vi "总磷总氮测量数据储存.vi"   [LabVIEW 2016, in "斯坦道总氮.lvlib"]
types:
  T1 = enum16{"水样测试", "标样核查", "跨度核查", "零点核查", "加标回收", "空白测试", "平行样"}
  T2 = cluster{"时间标识":timestamp, "测量模式":enum16{"维护数据", "水样测试", "标样核查", "零点核查", "跨度核查", "空白测试", "平行样测试", "加标回收", "空白校准", "标样校准", "初始化（清洗）", "快捷测试"}, "数据标记表":string, "监测值":sgl, "单位":u16, "数据标识":string, "因子编码":u32, "标样参考值":sgl, "F0":sgl, "F1":sgl, "F2":sgl, "F3":sgl, "F4":sgl, "F5":sgl, "F6":sgl, "F7":sgl, "X":sgl, "温度":sgl, "湿度":sgl, "量程标识":string, "SN":string, "跨度值":sgl, "X1":sgl}
  T3 = enum16{"维护数据", "水样测试", "标样核查", "零点核查", "跨度核查", "空白测试", "平行样测试", "加标回收", "空白校准", "标样校准", "初始化（清洗）", "快捷测试"}
  T4 = enum16{"维护数据", "水样测试", "标样核查", "零点核查", "跨度核查", "空白测试", "平行样测试", "加标回收", "空白校准", "标样校准", "初始化（清洗）"}
  T5 = cluster{"系统时间":timestamp, "工作状态":u16, "测量模式":enum16{"待机", "连续模式", "周期模式", "定点模式", "受控模式", "手动模式"}, "告警代码":u16, "故障代码":u16, "日志代码":u16, "软件版本":u16, "F0":sgl, "F1":sgl, "F2":sgl, "F3":sgl, "T":sgl, "H":sgl, "id":u16, "flowid":u16, "量程":u16, "总磷控温温度1":sgl, "营养盐控温温度2":sgl, "ADC":sgl}
  T6 = cluster{"运行模式":enum16{"维护模式", "常规模式", "应急模式", "质控模式"}, "质控频次":enum16{"关闭", "每天", "星期一", "星期二", "星期三", "星期四", "星期五", "星期六", "星期日"}, "空白核查时间":u16, "跨度核查时间":u16, "测量间隔":u16}
  T7 = cluster{"因子编码":u32, "单位":u16, "标样参考值":sgl, "水样数据时间":timestamp, "水样实测值":sgl, "水样数据标识":string, "标样数据时间":timestamp, "标样实测值":sgl, "标样数据标识":string, "空白数据时间":timestamp, "空白实测值":sgl, "空白数据标识":string, "零点核查数据时间":timestamp, "零点核查实测值":sgl, "零点核查数据标识":string, "跨度核查数据时间":timestamp, "跨度核查实测值":sgl, "跨度核查数据标识":string, "加标回收数据时间":timestamp, "加标回收实测值":sgl, "加标回收数据标识":string, "平行样数据时间":timestamp, "平行样实测值":sgl, "平行样数据标识":string, "F0":sgl, "F1":sgl, "F2":sgl, "F3":sgl, "F4":sgl, "F5":sgl, "F6":sgl, "F7":sgl, "温度":sgl, "湿度":sgl, "X值":sgl, "fidrange":u16, "X1值":sgl}[]
  T8 = cluster{"因子编码":u32, "单位":u16, "标样参考值":sgl, "水样数据时间":timestamp, "水样实测值":sgl, "水样数据标识":string, "标样数据时间":timestamp, "标样实测值":sgl, "标样数据标识":string, "空白数据时间":timestamp, "空白实测值":sgl, "空白数据标识":string, "零点核查数据时间":timestamp, "零点核查实测值":sgl, "零点核查数据标识":string, "跨度核查数据时间":timestamp, "跨度核查实测值":sgl, "跨度核查数据标识":string, "加标回收数据时间":timestamp, "加标回收实测值":sgl, "加标回收数据标识":string, "平行样数据时间":timestamp, "平行样实测值":sgl, "平行样数据标识":string, "F0":sgl, "F1":sgl, "F2":sgl, "F3":sgl, "F4":sgl, "F5":sgl, "F6":sgl, "F7":sgl, "温度":sgl, "湿度":sgl, "X值":sgl, "fidrange":u16, "X1值":sgl}
  T9 = cluster{"总磷跨度值":dbl, "总磷零点标准液浓度":dbl, "总磷跨度标准液浓度":dbl, "总磷标准液标准浓度":dbl, "总氮跨度值":dbl, "总氮零点标准液浓度":dbl, "总氮跨度标准液浓度":dbl, "总氮标准液标准浓度":dbl, "COD跨度值":dbl, "COD零点标准液浓度":dbl, "COD跨度标准液浓度":dbl, "COD标准液标准浓度":dbl, "氨氮跨度值":dbl, "氨氮零点标准液浓度":dbl, "氨氮跨度标准液浓度":dbl, "氨氮标准液标准浓度":dbl, "磷酸盐跨度值":dbl, "磷酸盐零点标准液浓度":dbl, "磷酸盐跨度标准液浓度":dbl, "磷酸盐标准液标准浓度":dbl, "硝氮跨度值":dbl, "硝氮零点标准液浓度":dbl, "硝氮跨度标准液浓度":dbl, "硝氮标准液标准浓度":dbl, "亚硝氮跨度值":dbl, "亚硝氮零点标准液浓度":dbl, "亚硝氮跨度标准液浓度":dbl, "亚硝氮标准液标准浓度":dbl, "硫化物跨度值":dbl, "硫化物零点标准液浓度":dbl, "硫化物跨度标准液浓度":dbl, "硫化物标准液标准浓度":dbl, "硅酸盐跨度值":dbl, "硅酸盐零点标准液浓度":dbl, "硅酸盐跨度标准液浓度":dbl, "硅酸盐标准液标准浓度":dbl, "总磷零点标准液偏差":dbl, "总磷跨度标准液偏差":dbl, "总磷标准液标准偏差":dbl, "总氮零点标准液偏差":dbl, "总氮跨度标准液偏差":dbl, "总氮标准液标准偏差":dbl, "COD零点标准液偏差":dbl, "COD跨度标准液偏差":dbl, "COD标准液标准偏差":dbl, "氨氮零点标准液偏差":dbl, "氨氮跨度标准液偏差":dbl, "氨氮标准液标准偏差":dbl, "磷酸盐零点标准液偏差":dbl, "磷酸盐跨度标准液偏差":dbl, "磷酸盐标准液标准偏差":dbl, "硝氮零点标准液偏差":dbl, "硝氮跨度标准液偏差":dbl, "硝氮标准液标准偏差":dbl, "亚硝氮零点标准液偏差":dbl, "亚硝氮跨度标准液偏差":dbl, "亚硝氮标准液标准偏差":dbl, "硫化物零点标准液偏差":dbl, "硫化物跨度标准液偏差":dbl, "硫化物标准液标准偏差":dbl, "硅酸盐零点标准液偏差":dbl, "硅酸盐跨度标准液偏差":dbl, "硅酸盐标准液标准偏差":dbl, "氟化物跨度值":dbl, "氟化物零点标准液浓度":dbl, "氟化物跨度标准液浓度":dbl, "氟化物标准液标准浓度":dbl, "氟化物零点标准液偏差":dbl, "氟化物跨度标准液偏差":dbl, "氟化物标准液标准偏差":dbl}
  T10 = typedef "斯坦道总氮.lvlib/关键参数.ctl" = cluster{"测量量程":sgl, "测量检出限":sgl, "测量精度":sgl, "测量间隔":sgl, "消解温度":sgl, "消解时长":sgl, "三项式系数":sgl, "二次多项式系数":sgl, "曲线斜率":sgl, "曲线截距":sgl, "线性相关系数":sgl, "空白校准时间":timestamp, "标样校准时间":timestamp, "测量信号值":sgl, "稀释倍数":sgl, "空白标定系数":sgl, "量程系数":sgl}
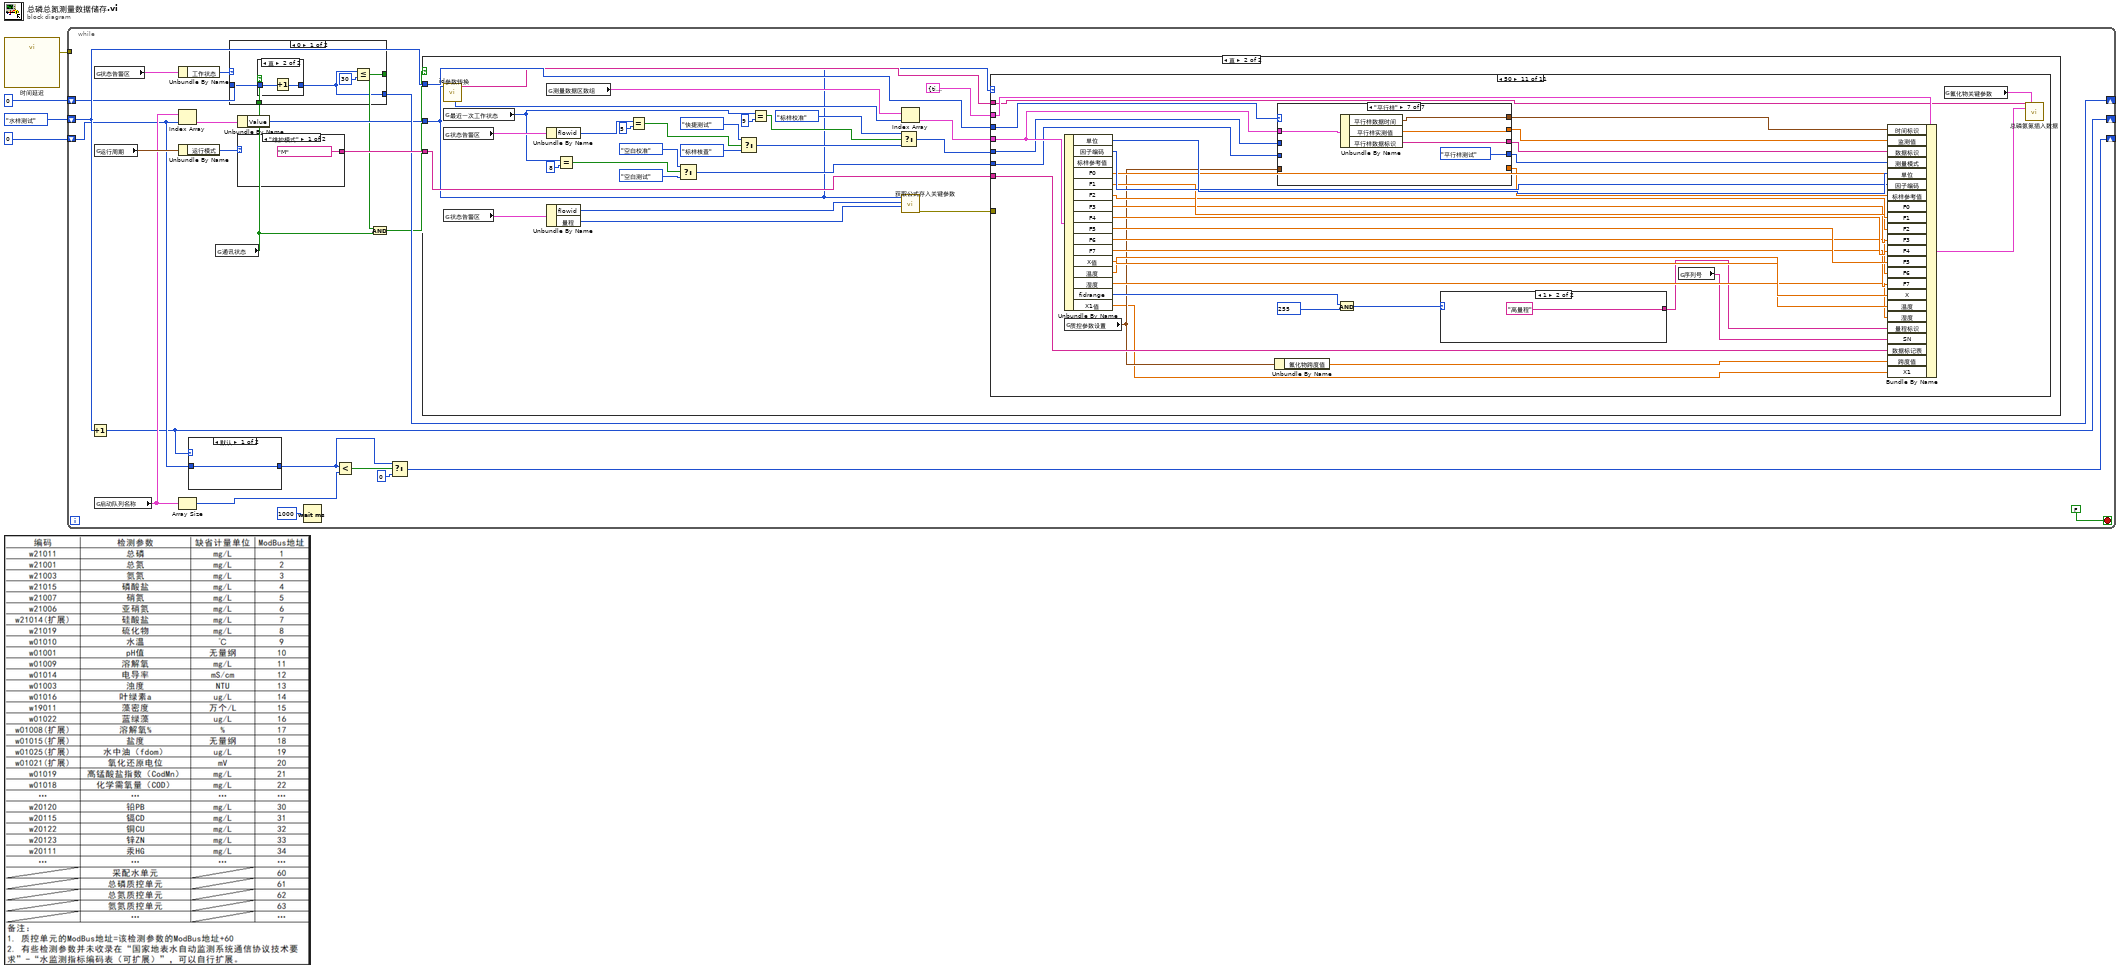
[diagram p0: block diagram]
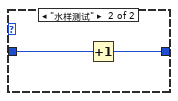
[diagram p2: hidden frame]
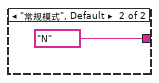
[diagram p5: hidden frame]
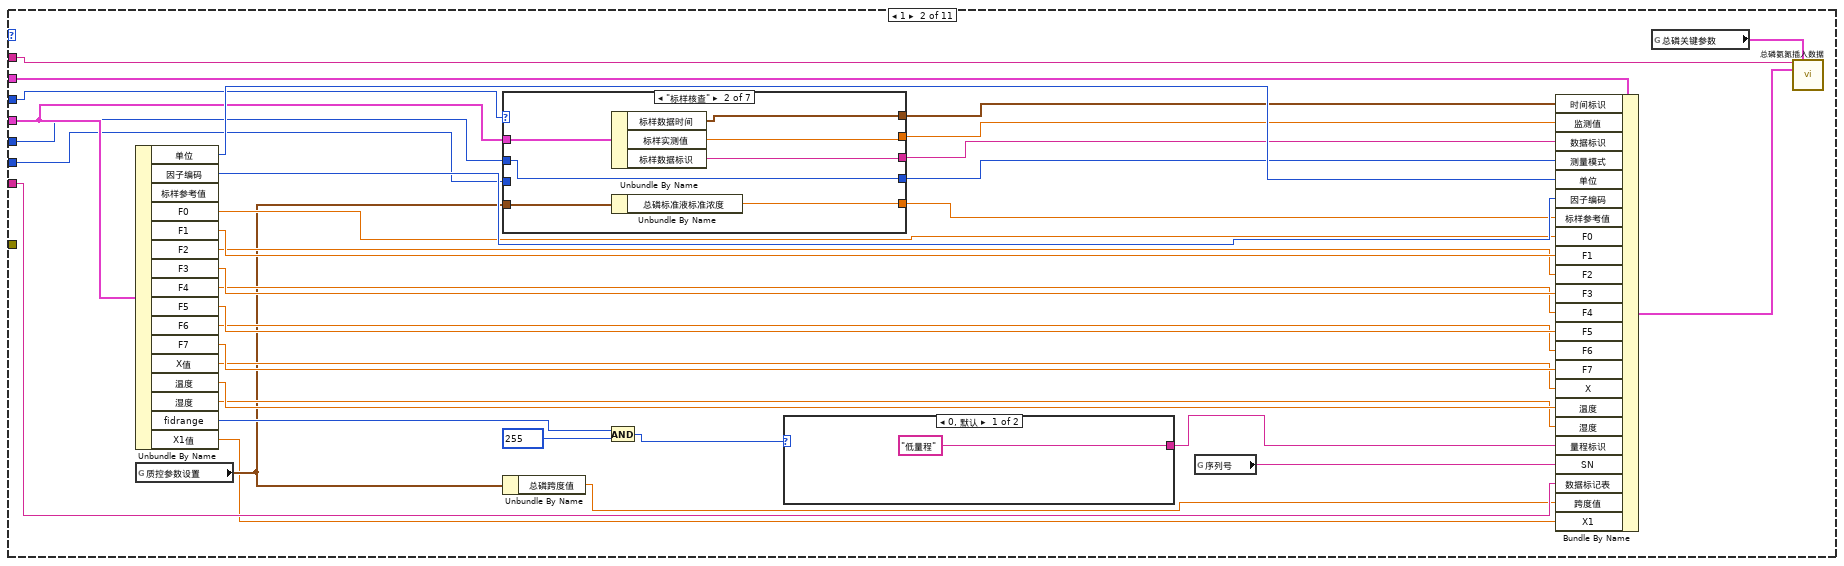
[diagram p8: hidden frame]
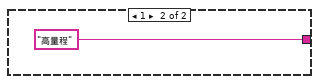
[diagram p9: hidden frame]
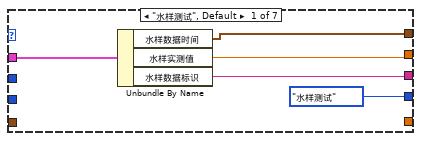
[diagram p10: hidden frame]
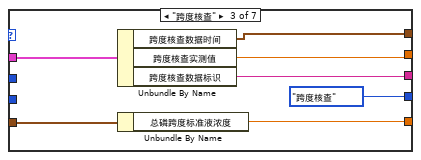
[diagram p11: hidden frame]
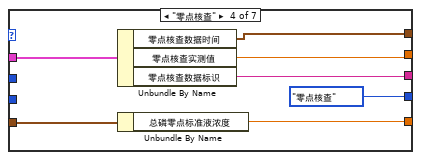
[diagram p12: hidden frame]
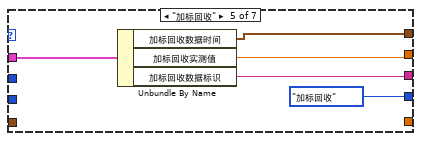
[diagram p13: hidden frame]
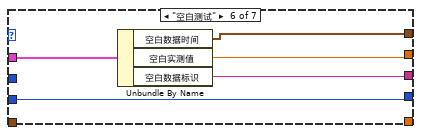
[diagram p14: hidden frame]
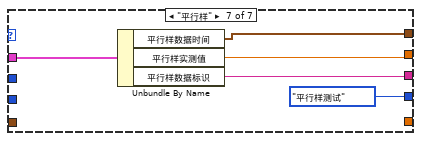
[diagram p15: hidden frame]
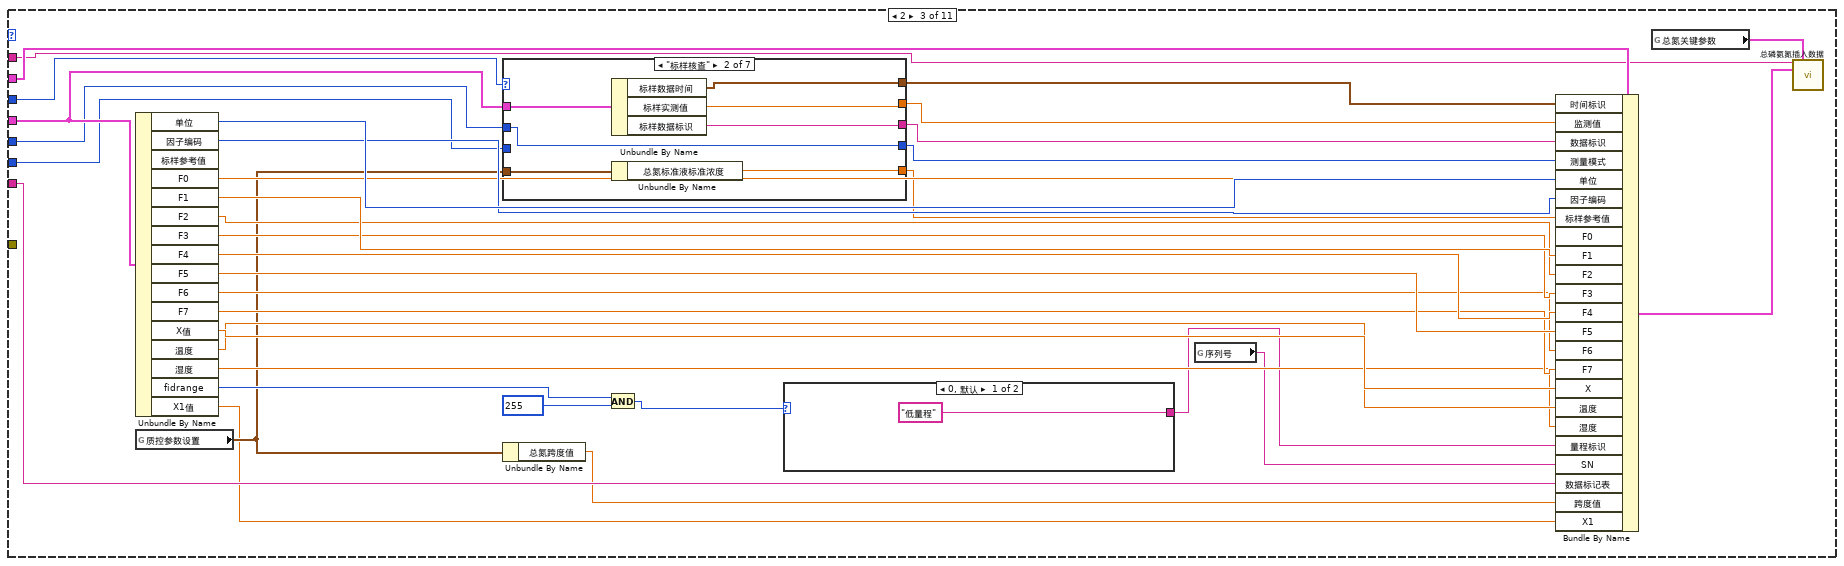
[diagram p16: hidden frame]
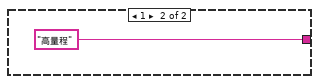
[diagram p17: hidden frame]
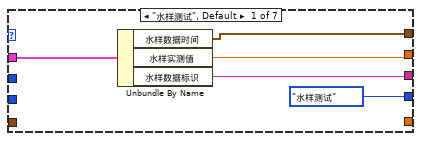
[diagram p18: hidden frame]
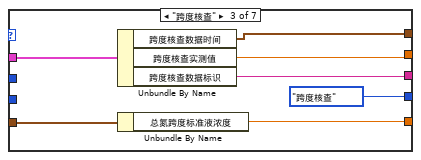
[diagram p19: hidden frame]
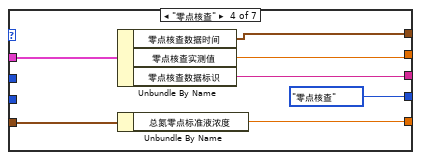
[diagram p20: hidden frame]
diagram:
  n1 = call "时间延迟"() -> ("error out"=w2:errorcluster)  [unwired: 11 in]
  n2 = while {
    shift-right: [w10] -> _
    shift-left: T1."水样测试" ("测量模式") -> [w25]
    shift-right: [w19] -> _
    shift-left: u32 0 ("等待时间（毫秒）") -> [w20]
    tunnel: w2 -> [_]
    shift-right: [w11] -> _
    shift-left: 0 -> [w14]
    stop <- FALSE stop-if-true
    n3 = Increment(x=w25) -> (x+1=w10:T1)
    n4 = global read "VAR总磷总氮全局变量.vi" "状态告警区"() -> (w22:T5)
    n5 = global read "总磷总氮断电保存全局变量.vi" "运行周期"() -> (w24:T6)
    n6 = global read "model config var.vi" "启动队列名称"() -> (w15:cluster{"String":string, "Value":u16}[])
    n7 = Unbundle By Name(w22) -> ("工作状态"=w21:u16)
    n8 = Index Array(array=w15, index=w14) -> (element=w17:cluster{"String":string, "Value":u16})
    n9 = Unbundle By Name(w24) -> ("运行模式"=w23:enum16{"维护模式", "常规模式", "应急模式", "质控模式"})
    n10 = Array Size(array=w15) -> (size(s)=w13:i32)
    n11 = case shown="默认" w10 {
      tunnel: w14 -> [w28 w30]
      tunnel: [w28 w29] -> w8
      frame Default {
      }
      frame "水样测试" {
        n12 = Increment(x=w30) -> (x+1=w29:i32)
      }
    }
    n13 = global read "VAR总磷总氮全局变量.vi" "通讯状态"() -> (w5:bool)
    n14 = case shown="0" w21 {
      tunnel: w20 -> [w35 _]
      tunnel: [w34 _] -> w19
      tunnel: [w32 _] -> w7
      tunnel: w5 -> [w31 _]
      frame 0 {
        n15 = case shown="真" w31 {
          tunnel: w35 -> [_ w37]
          tunnel: [_ w36] -> w34
          frame False {
          }
          frame True {
            n16 = Increment(x=w37) -> (x+1=w36:u32)
          }
        }
        n17 = Less Or Equal?(x=w34, y=u32 30) -> (x <= y?=w32:bool)
      }
      frame 1, Default {
      }
    }
    n18 = Unbundle By Name(w17) -> ("Value"=w16:u16)
    n19 = case shown="\"维护模式\"" w23 {
      tunnel: ["M" ("数据标记表") "N" ("数据标记表")] -> w26
      frame "维护模式" {
      }
      frame "常规模式", Default {
      }
    }
    n20 = Wait (ms)(milliseconds to wait=u32 1000 ("等待时间（毫秒）")) -> ()  [unwired: 1 out]
    n21 = Less?(x=w8, y=w13) -> (x < y?=w12:bool)
    n22 = And(x=w7, y=w5) -> (x .and. y?=w6:bool)
    n23 = Select(t=w8, s=w12, f=0) -> (s? t:f=w11:i32)
    n24 = case shown="真" w6 {
      tunnel: w26 -> [_ w68]
      tunnel: w25 -> [_ w67]
      tunnel: w16 -> [_ w40]
      frame False {
      }
      frame True {
        n25 = call "id参数转换.vi"("id"=w40) -> ("table输出"=w63:string, "数组资源索引"=w62:i32)  [unwired: 9 in]
        n26 = global read "VAR总磷总氮全局变量.vi" "最近一次工作状态"() -> (w54:u16)
        n27 = global read "VAR总磷总氮全局变量.vi" "状态告警区"() -> (w66:T5)
        n28 = global read "VAR总磷总氮全局变量.vi" "状态告警区"() -> (w44:T5)
        n29 = global read "VAR总磷总氮全局变量.vi" "测量数据区数组"() -> (w65:T7)
        n30 = Unbundle By Name(w66) -> ("flowid"=w51:u16)
        n31 = Unbundle By Name(w44) -> ("flowid"=w43:u16, "量程"=w42:u16)
        n32 = Equal?(x=w54, y=u16 8) -> (x = y?=w60:bool)
        n33 = Equal?(x=w51, y=u16 5) -> (x = y?=w49:bool)
        n34 = Select(t=T3."空白校准" ("测量模式"), s=w60, f=T3."空白测试" ("测量模式")) -> (s? t:f=w53:T3)
        n35 = Select(t=T3."快捷测试" ("测量模式"), s=w49, f=T3."标样核查" ("测量模式")) -> (s? t:f=w46:T3)
        n36 = Equal?(x=w54, y=u16 9) -> (x = y?=w56:bool)
        n37 = Select(t=T3."标样校准" ("测量模式"), s=w56, f=w46) -> (s? t:f=w52:T3)
        n38 = Index Array(array=w65, index=w62) -> (element=w64:T8)
        n39 = call "获取公式存入关键参数.vi"("量程"=w42, "flowid"=w43, "id"=w40) -> ("error out"=w41:errorcluster)  [unwired: 8 in]
        n40 = case shown="50" w40 {
          tunnel: w68 -> [_ w79 w157 w236 w314 w392 w470 w548 w626 w704 w782]
          tunnel: w67 -> [_ w87 w168 w246 w324 w402 w480 w558 w636 w714 w792]
          tunnel: T2 {"时间标识"=timestamp(0 s since 1904-01-01), "测量模式"=enum."水样测试", "数据标记表"="N", "监测值"=0.0, "单位"=0, "数据标识"="", "因子编码"=0, "标样参考值"=0.0, "F0"=0.0, "F1"=0.0, "F2"=0.0, "F3"=0.0, "F4"=0.0, "F5"=0.0, "F6"=0.0, "F7"=0.0, "X"=0.0, "温度"=0.0, "湿度"=0.0, "量程标识"="", "SN"="", "跨度值"=0.0, "X1"=0.0} ("data") -> [_ w77 w155 w234 w312 w390 w468 w546 w624 w702 w780]
          tunnel: w64 -> [_ w74 w152 w231 w309 w387 w465 w543 w621 w698 w776]
          tunnel: w63 -> [_ w73 w151 w229 w307 w385 w463 w541 w619 w697 w775]
          tunnel: w53 -> [_ w72 w150 w227 w306 w384 w462 w539 w618 w696 w774]
          tunnel: w52 -> [_ w71 w149 w228 w305 w383 w461 w540 w617 w695 w773]
          tunnel: w41 -> [_ _ _ _ _ _ _ _ _ _ _]
          frame Default {
          }
          frame 1 {
            n41 = Unbundle By Name(w74) -> ("单位"=w103:u16, "因子编码"=w102:u32, "F0"=w101:sgl, "F1"=w100:sgl, "F2"=w99:sgl, "F3"=w98:sgl, "F4"=w97:sgl, "F5"=w96:sgl, "F6"=w95:sgl, "F7"=w94:sgl, "X值"=w93:sgl, "温度"=w92:sgl, "湿度"=w91:sgl, "fidrange"=w85:u16, "X1值"=w69:sgl)  [unwired: 1 out]
            n42 = global read "总磷总氮断电保存全局变量.vi" "质控参数设置"() -> (w76:T9)
            n43 = case shown="\"标样核查\"" w87 {
              tunnel: w74 -> [w110 w117 w124 w131 w136 w141 w146]
              tunnel: [w109 w116 w123 w130 w135 w140 w145] -> w88
              tunnel: [w108 w115 w122 w129 w134 w139 w144] -> w89
              tunnel: [w107 w114 w121 w128 w133 w138 w143] -> w90
              tunnel: [T4."水样测试" ("测量模式") w111 T4."跨度核查" ("测量模式") T4."零点核查" ("测量模式") T4."加标回收" ("测量模式") w137 T4."平行样测试" ("测量模式")] -> w78
              tunnel: w76 -> [_ w113 w119 w126 _ _ _]
              tunnel: [_ w112 w118 w125 _ _ _] -> w86
              tunnel: w72 -> [_ _ _ _ _ w137 _]
              tunnel: w71 -> [_ w111 _ _ _ _ _]
              frame "水样测试", Default {
                n44 = Unbundle By Name(w110) -> ("水样数据时间"=w109:timestamp, "水样实测值"=w108:sgl, "水样数据标识"=w107:string)
              }
              frame "标样核查" {
                n45 = Unbundle By Name(w117) -> ("标样数据时间"=w116:timestamp, "标样实测值"=w115:sgl, "标样数据标识"=w114:string)
                n46 = Unbundle By Name(w113) -> ("总磷标准液标准浓度"=w112:dbl)
              }
              frame "跨度核查" {
                n47 = Unbundle By Name(w124) -> ("跨度核查数据时间"=w123:timestamp, "跨度核查实测值"=w122:sgl, "跨度核查数据标识"=w121:string)
                n48 = Unbundle By Name(w119) -> ("总磷跨度标准液浓度"=w118:dbl)
              }
              frame "零点核查" {
                n49 = Unbundle By Name(w131) -> ("零点核查数据时间"=w130:timestamp, "零点核查实测值"=w129:sgl, "零点核查数据标识"=w128:string)
                n50 = Unbundle By Name(w126) -> ("总磷零点标准液浓度"=w125:dbl)
              }
              frame "加标回收" {
                n51 = Unbundle By Name(w136) -> ("加标回收数据时间"=w135:timestamp, "加标回收实测值"=w134:sgl, "加标回收数据标识"=w133:string)
              }
              frame "空白测试" {
                n52 = Unbundle By Name(w141) -> ("空白数据时间"=w140:timestamp, "空白实测值"=w139:sgl, "空白数据标识"=w138:string)
              }
              frame "平行样" {
                n53 = Unbundle By Name(w146) -> ("平行样数据时间"=w145:timestamp, "平行样实测值"=w144:sgl, "平行样数据标识"=w143:string)
              }
            }
            n54 = Unbundle By Name(w76) -> ("总磷跨度值"=w75:dbl)
            n55 = And(x=w85, y=u16 255) -> (x .and. y?=w83:u16)
            n56 = case shown="0, 默认" w83 {
              tunnel: ["低量程" ("格式字符串") "高量程" ("格式字符串")] -> w82
              frame 0, Default {
              }
              frame 1 {
              }
            }
            n57 = global read "VAR总磷总氮全局变量.vi" "序列号"() -> (w80:string)
            n58 = Bundle By Name(cluster=w77, "时间标识"=w88, "监测值"=w89, "数据标识"=w90, "测量模式"=w78, "单位"=w103, "因子编码"=w102, "标样参考值"=w86, "F0"=w101, "F1"=w100, "F2"=w99, "F3"=w98, "F4"=w97, "F5"=w96, "F6"=w95, "F7"=w94, "X"=w93, "温度"=w92, "湿度"=w91, "量程标识"=w82, "SN"=w80, "数据标记表"=w79, "跨度值"=w75, "X1"=w69) -> (w81:T2)
            n59 = global read "VAR总磷总氮全局变量.vi" "总磷关键参数"() -> (w70:T10)
            n60 = call "总磷氨氮插入数据.vi"("table"=w73, "关键参数"=w70, "data"=w81) -> ()  [unwired: 12 in, 1 out]
          }
          frame 2 {
            n61 = Unbundle By Name(w152) -> ("单位"=w181:u16, "因子编码"=w180:u32, "F0"=w179:sgl, "F1"=w178:sgl, "F2"=w177:sgl, "F3"=w176:sgl, "F4"=w175:sgl, "F5"=w174:sgl, "F6"=w173:sgl, "F7"=w172:sgl, "X值"=w171:sgl, "温度"=w170:sgl, "湿度"=w169:sgl, "fidrange"=w161:u16, "X1值"=w147:sgl)  [unwired: 1 out]
            n62 = global read "总磷总氮断电保存全局变量.vi" "质控参数设置"() -> (w154:T9)
            n63 = case shown="\"标样核查\"" w168 {
              tunnel: w152 -> [w188 w195 w202 w209 w214 w219 w224]
              tunnel: [w187 w194 w201 w208 w213 w218 w223] -> w167
              tunnel: [w186 w193 w200 w207 w212 w217 w222] -> w166
              tunnel: [w185 w192 w199 w206 w211 w216 w221] -> w165
              tunnel: [T4."水样测试" ("测量模式") w189 T4."跨度核查" ("测量模式") T4."零点核查" ("测量模式") T4."加标回收" ("测量模式") w215 T4."平行样测试" ("测量模式")] -> w156
              tunnel: w154 -> [_ w191 w197 w204 _ _ _]
              tunnel: [_ w190 w196 w203 _ _ _] -> w164
              tunnel: w150 -> [_ _ _ _ _ w215 _]
              tunnel: w149 -> [_ w189 _ _ _ _ _]
              frame "水样测试", Default {
                n64 = Unbundle By Name(w188) -> ("水样数据时间"=w187:timestamp, "水样实测值"=w186:sgl, "水样数据标识"=w185:string)
              }
              frame "标样核查" {
                n65 = Unbundle By Name(w195) -> ("标样数据时间"=w194:timestamp, "标样实测值"=w193:sgl, "标样数据标识"=w192:string)
                n66 = Unbundle By Name(w191) -> ("总氮标准液标准浓度"=w190:dbl)
              }
              frame "跨度核查" {
                n67 = Unbundle By Name(w202) -> ("跨度核查数据时间"=w201:timestamp, "跨度核查实测值"=w200:sgl, "跨度核查数据标识"=w199:string)
                n68 = Unbundle By Name(w197) -> ("总氮跨度标准液浓度"=w196:dbl)
              }
              frame "零点核查" {
                n69 = Unbundle By Name(w209) -> ("零点核查数据时间"=w208:timestamp, "零点核查实测值"=w207:sgl, "零点核查数据标识"=w206:string)
                n70 = Unbundle By Name(w204) -> ("总氮零点标准液浓度"=w203:dbl)
              }
              frame "加标回收" {
                n71 = Unbundle By Name(w214) -> ("加标回收数据时间"=w213:timestamp, "加标回收实测值"=w212:sgl, "加标回收数据标识"=w211:string)
              }
              frame "空白测试" {
                n72 = Unbundle By Name(w219) -> ("空白数据时间"=w218:timestamp, "空白实测值"=w217:sgl, "空白数据标识"=w216:string)
              }
              frame "平行样" {
                n73 = Unbundle By Name(w224) -> ("平行样数据时间"=w223:timestamp, "平行样实测值"=w222:sgl, "平行样数据标识"=w221:string)
              }
            }
            n74 = Unbundle By Name(w154) -> ("总氮跨度值"=w153:dbl)
            n75 = And(x=w161, y=u16 255) -> (x .and. y?=w162:u16)
            n76 = case shown="0, 默认" w162 {
              tunnel: ["低量程" ("格式字符串") "高量程" ("格式字符串")] -> w160
              frame 0, Default {
              }
              frame 1 {
              }
            }
            n77 = global read "VAR总磷总氮全局变量.vi" "序列号"() -> (w158:string)
            n78 = Bundle By Name(cluster=w155, "时间标识"=w167, "监测值"=w166, "数据标识"=w165, "测量模式"=w156, "单位"=w181, "因子编码"=w180, "标样参考值"=w164, "F0"=w179, "F1"=w178, "F2"=w177, "F3"=w176, "F4"=w175, "F5"=w174, "F6"=w173, "F7"=w172, "X"=w171, "温度"=w170, "湿度"=w169, "量程标识"=w160, "SN"=w158, "数据标记表"=w157, "跨度值"=w153, "X1"=w147) -> (w159:T2)
            n79 = global read "VAR总磷总氮全局变量.vi" "总氮关键参数"() -> (w148:T10)
            n80 = call "总磷氨氮插入数据.vi"("table"=w151, "关键参数"=w148, "data"=w159) -> ()  [unwired: 12 in, 1 out]
          }
          frame 3 {
            n81 = Unbundle By Name(w231) -> ("单位"=w259:u16, "因子编码"=w258:u32, "F0"=w257:sgl, "F1"=w256:sgl, "F2"=w255:sgl, "F3"=w254:sgl, "F4"=w253:sgl, "F5"=w252:sgl, "F6"=w251:sgl, "F7"=w250:sgl, "X值"=w249:sgl, "温度"=w248:sgl, "湿度"=w247:sgl, "fidrange"=w239:u16, "X1值"=w225:sgl)  [unwired: 1 out]
            n82 = global read "总磷总氮断电保存全局变量.vi" "质控参数设置"() -> (w233:T9)
            n83 = case shown="\"空白测试\"" w246 {
              tunnel: w231 -> [w266 w273 w280 w287 w292 w297 w302]
              tunnel: [w265 w272 w279 w286 w291 w296 w301] -> w245
              tunnel: [w264 w271 w278 w285 w290 w295 w300] -> w244
              tunnel: [w263 w270 w277 w284 w289 w294 w299] -> w243
              tunnel: [T4."水样测试" ("测量模式") w267 T4."跨度核查" ("测量模式") T4."零点核查" ("测量模式") T4."加标回收" ("测量模式") w293 T4."平行样测试" ("测量模式")] -> w235
              tunnel: w233 -> [_ w269 w275 w282 _ _ _]
              tunnel: [_ w268 w274 w281 _ _ _] -> w242
              tunnel: w228 -> [_ w267 _ _ _ _ _]
              tunnel: w227 -> [_ _ _ _ _ w293 _]
              frame "水样测试", Default {
                n84 = Unbundle By Name(w266) -> ("水样数据时间"=w265:timestamp, "水样实测值"=w264:sgl, "水样数据标识"=w263:string)
              }
              frame "标样核查" {
                n85 = Unbundle By Name(w273) -> ("标样数据时间"=w272:timestamp, "标样实测值"=w271:sgl, "标样数据标识"=w270:string)
                n86 = Unbundle By Name(w269) -> ("氨氮标准液标准浓度"=w268:dbl)
              }
              frame "跨度核查" {
                n87 = Unbundle By Name(w280) -> ("跨度核查数据时间"=w279:timestamp, "跨度核查实测值"=w278:sgl, "跨度核查数据标识"=w277:string)
                n88 = Unbundle By Name(w275) -> ("氨氮跨度标准液浓度"=w274:dbl)
              }
              frame "零点核查" {
                n89 = Unbundle By Name(w287) -> ("零点核查数据时间"=w286:timestamp, "零点核查实测值"=w285:sgl, "零点核查数据标识"=w284:string)
                n90 = Unbundle By Name(w282) -> ("氨氮零点标准液浓度"=w281:dbl)
              }
              frame "加标回收" {
                n91 = Unbundle By Name(w292) -> ("加标回收数据时间"=w291:timestamp, "加标回收实测值"=w290:sgl, "加标回收数据标识"=w289:string)
              }
              frame "空白测试" {
                n92 = Unbundle By Name(w297) -> ("空白数据时间"=w296:timestamp, "空白实测值"=w295:sgl, "空白数据标识"=w294:string)
              }
              frame "平行样" {
                n93 = Unbundle By Name(w302) -> ("平行样数据时间"=w301:timestamp, "平行样实测值"=w300:sgl, "平行样数据标识"=w299:string)
              }
            }
            n94 = Unbundle By Name(w233) -> ("氨氮跨度值"=w232:dbl)
            n95 = And(x=w239, y=u16 255) -> (x .and. y?=w240:u16)
            n96 = case shown="0, 默认" w240 {
              tunnel: ["低量程" ("格式字符串") "高量程" ("格式字符串")] -> w238
              frame 0, Default {
              }
              frame 1 {
              }
            }
            n97 = global read "VAR总磷总氮全局变量.vi" "序列号"() -> (w237:string)
            n98 = Bundle By Name(cluster=w234, "时间标识"=w245, "监测值"=w244, "数据标识"=w243, "测量模式"=w235, "单位"=w259, "因子编码"=w258, "标样参考值"=w242, "F0"=w257, "F1"=w256, "F2"=w255, "F3"=w254, "F4"=w253, "F5"=w252, "F6"=w251, "F7"=w250, "X"=w249, "温度"=w248, "湿度"=w247, "量程标识"=w238, "SN"=w237, "数据标记表"=w236, "跨度值"=w232, "X1"=w225) -> (w230:T2)
            n99 = global read "VAR总磷总氮全局变量.vi" "氨氮关键参数"() -> (w226:T10)
            n100 = call "总磷氨氮插入数据.vi"("table"=w229, "关键参数"=w226, "data"=w230) -> ()  [unwired: 12 in, 1 out]
          }
          frame 4 {
            n101 = Unbundle By Name(w309) -> ("单位"=w337:u16, "因子编码"=w336:u32, "F0"=w335:sgl, "F1"=w334:sgl, "F2"=w333:sgl, "F3"=w332:sgl, "F4"=w331:sgl, "F5"=w330:sgl, "F6"=w329:sgl, "F7"=w328:sgl, "X值"=w327:sgl, "温度"=w326:sgl, "湿度"=w325:sgl, "fidrange"=w317:u16, "X1值"=w303:sgl)  [unwired: 1 out]
            n102 = global read "总磷总氮断电保存全局变量.vi" "质控参数设置"() -> (w311:T9)
            n103 = case shown="\"标样核查\"" w324 {
              tunnel: w309 -> [w344 w351 w358 w365 w370 w375 w380]
              tunnel: [w343 w350 w357 w364 w369 w374 w379] -> w323
              tunnel: [w342 w349 w356 w363 w368 w373 w378] -> w322
              tunnel: [w341 w348 w355 w362 w367 w372 w377] -> w321
              tunnel: [T4."水样测试" ("测量模式") w345 T4."跨度核查" ("测量模式") T4."零点核查" ("测量模式") T4."加标回收" ("测量模式") w371 T4."平行样测试" ("测量模式")] -> w313
              tunnel: w311 -> [_ w347 w353 w360 _ _ _]
              tunnel: [_ w346 w352 w359 _ _ _] -> w320
              tunnel: w306 -> [_ _ _ _ _ w371 _]
              tunnel: w305 -> [_ w345 _ _ _ _ _]
              frame "水样测试", Default {
                n104 = Unbundle By Name(w344) -> ("水样数据时间"=w343:timestamp, "水样实测值"=w342:sgl, "水样数据标识"=w341:string)
              }
              frame "标样核查" {
                n105 = Unbundle By Name(w351) -> ("标样数据时间"=w350:timestamp, "标样实测值"=w349:sgl, "标样数据标识"=w348:string)
                n106 = Unbundle By Name(w347) -> ("磷酸盐标准液标准浓度"=w346:dbl)
              }
              frame "跨度核查" {
                n107 = Unbundle By Name(w358) -> ("跨度核查数据时间"=w357:timestamp, "跨度核查实测值"=w356:sgl, "跨度核查数据标识"=w355:string)
                n108 = Unbundle By Name(w353) -> ("磷酸盐跨度标准液浓度"=w352:dbl)
              }
              frame "零点核查" {
                n109 = Unbundle By Name(w365) -> ("零点核查数据时间"=w364:timestamp, "零点核查实测值"=w363:sgl, "零点核查数据标识"=w362:string)
                n110 = Unbundle By Name(w360) -> ("磷酸盐零点标准液浓度"=w359:dbl)
              }
              frame "加标回收" {
                n111 = Unbundle By Name(w370) -> ("加标回收数据时间"=w369:timestamp, "加标回收实测值"=w368:sgl, "加标回收数据标识"=w367:string)
              }
              frame "空白测试" {
                n112 = Unbundle By Name(w375) -> ("空白数据时间"=w374:timestamp, "空白实测值"=w373:sgl, "空白数据标识"=w372:string)
              }
              frame "平行样" {
                n113 = Unbundle By Name(w380) -> ("平行样数据时间"=w379:timestamp, "平行样实测值"=w378:sgl, "平行样数据标识"=w377:string)
              }
            }
            n114 = Unbundle By Name(w311) -> ("磷酸盐跨度值"=w310:dbl)
            n115 = And(x=w317, y=u16 255) -> (x .and. y?=w318:u16)
            n116 = case shown="0, 默认" w318 {
              tunnel: ["低量程" ("格式字符串") "高量程" ("格式字符串")] -> w316
              frame 0, Default {
              }
              frame 1 {
              }
            }
            n117 = global read "VAR总磷总氮全局变量.vi" "序列号"() -> (w315:string)
            n118 = Bundle By Name(cluster=w312, "时间标识"=w323, "监测值"=w322, "数据标识"=w321, "测量模式"=w313, "单位"=w337, "因子编码"=w336, "标样参考值"=w320, "F0"=w335, "F1"=w334, "F2"=w333, "F3"=w332, "F4"=w331, "F5"=w330, "F6"=w329, "F7"=w328, "X"=w327, "温度"=w326, "湿度"=w325, "量程标识"=w316, "SN"=w315, "数据标记表"=w314, "跨度值"=w310, "X1"=w303) -> (w308:T2)
            n119 = global read "VAR总磷总氮全局变量.vi" "磷酸盐关键参数"() -> (w304:T10)
            n120 = call "总磷氨氮插入数据.vi"("table"=w307, "关键参数"=w304, "data"=w308) -> ()  [unwired: 12 in, 1 out]
          }
          frame 5 {
            n121 = Unbundle By Name(w387) -> ("单位"=w415:u16, "因子编码"=w414:u32, "F0"=w413:sgl, "F1"=w412:sgl, "F2"=w411:sgl, "F3"=w410:sgl, "F4"=w409:sgl, "F5"=w408:sgl, "F6"=w407:sgl, "F7"=w406:sgl, "X值"=w405:sgl, "温度"=w404:sgl, "湿度"=w403:sgl, "fidrange"=w395:u16, "X1值"=w381:sgl)  [unwired: 1 out]
            n122 = global read "总磷总氮断电保存全局变量.vi" "质控参数设置"() -> (w389:T9)
            n123 = case shown="\"标样核查\"" w402 {
              tunnel: w387 -> [w422 w429 w436 w443 w448 w453 w458]
              tunnel: [w421 w428 w435 w442 w447 w452 w457] -> w401
              tunnel: [w420 w427 w434 w441 w446 w451 w456] -> w400
              tunnel: [w419 w426 w433 w440 w445 w450 w455] -> w399
              tunnel: [T4."水样测试" ("测量模式") w423 T4."跨度核查" ("测量模式") T4."零点核查" ("测量模式") T4."加标回收" ("测量模式") w449 T4."平行样测试" ("测量模式")] -> w391
              tunnel: w389 -> [_ w425 w431 w438 _ _ _]
              tunnel: [_ w424 w430 w437 _ _ _] -> w398
              tunnel: w384 -> [_ _ _ _ _ w449 _]
              tunnel: w383 -> [_ w423 _ _ _ _ _]
              frame "水样测试", Default {
                n124 = Unbundle By Name(w422) -> ("水样数据时间"=w421:timestamp, "水样实测值"=w420:sgl, "水样数据标识"=w419:string)
              }
              frame "标样核查" {
                n125 = Unbundle By Name(w429) -> ("标样数据时间"=w428:timestamp, "标样实测值"=w427:sgl, "标样数据标识"=w426:string)
                n126 = Unbundle By Name(w425) -> ("硝氮标准液标准浓度"=w424:dbl)
              }
              frame "跨度核查" {
                n127 = Unbundle By Name(w436) -> ("跨度核查数据时间"=w435:timestamp, "跨度核查实测值"=w434:sgl, "跨度核查数据标识"=w433:string)
                n128 = Unbundle By Name(w431) -> ("硝氮跨度标准液浓度"=w430:dbl)
              }
              frame "零点核查" {
                n129 = Unbundle By Name(w443) -> ("零点核查数据时间"=w442:timestamp, "零点核查实测值"=w441:sgl, "零点核查数据标识"=w440:string)
                n130 = Unbundle By Name(w438) -> ("硝氮零点标准液浓度"=w437:dbl)
              }
              frame "加标回收" {
                n131 = Unbundle By Name(w448) -> ("加标回收数据时间"=w447:timestamp, "加标回收实测值"=w446:sgl, "加标回收数据标识"=w445:string)
              }
              frame "空白测试" {
                n132 = Unbundle By Name(w453) -> ("空白数据时间"=w452:timestamp, "空白实测值"=w451:sgl, "空白数据标识"=w450:string)
              }
              frame "平行样" {
                n133 = Unbundle By Name(w458) -> ("平行样数据时间"=w457:timestamp, "平行样实测值"=w456:sgl, "平行样数据标识"=w455:string)
              }
            }
            n134 = Unbundle By Name(w389) -> ("硝氮跨度值"=w388:dbl)
            n135 = And(x=w395, y=u16 255) -> (x .and. y?=w396:u16)
            n136 = case shown="0, 默认" w396 {
              tunnel: ["低量程" ("格式字符串") "高量程" ("格式字符串")] -> w394
              frame 0, Default {
              }
              frame 1 {
              }
            }
            n137 = global read "VAR总磷总氮全局变量.vi" "序列号"() -> (w393:string)
            n138 = Bundle By Name(cluster=w390, "时间标识"=w401, "监测值"=w400, "数据标识"=w399, "测量模式"=w391, "单位"=w415, "因子编码"=w414, "标样参考值"=w398, "F0"=w413, "F1"=w412, "F2"=w411, "F3"=w410, "F4"=w409, "F5"=w408, "F6"=w407, "F7"=w406, "X"=w405, "温度"=w404, "湿度"=w403, "量程标识"=w394, "SN"=w393, "数据标记表"=w392, "跨度值"=w388, "X1"=w381) -> (w386:T2)
            n139 = global read "VAR总磷总氮全局变量.vi" "硝氮关键参数"() -> (w382:T10)
            n140 = call "总磷氨氮插入数据.vi"("table"=w385, "关键参数"=w382, "data"=w386) -> ()  [unwired: 12 in, 1 out]
          }
          frame 6 {
            n141 = Unbundle By Name(w465) -> ("单位"=w493:u16, "因子编码"=w492:u32, "F0"=w491:sgl, "F1"=w490:sgl, "F2"=w489:sgl, "F3"=w488:sgl, "F4"=w487:sgl, "F5"=w486:sgl, "F6"=w485:sgl, "F7"=w484:sgl, "X值"=w483:sgl, "温度"=w482:sgl, "湿度"=w481:sgl, "fidrange"=w473:u16, "X1值"=w459:sgl)  [unwired: 1 out]
            n142 = global read "总磷总氮断电保存全局变量.vi" "质控参数设置"() -> (w467:T9)
            n143 = case shown="\"标样核查\"" w480 {
              tunnel: w465 -> [w500 w507 w514 w521 w526 w531 w536]
              tunnel: [w499 w506 w513 w520 w525 w530 w535] -> w479
              tunnel: [w498 w505 w512 w519 w524 w529 w534] -> w478
              tunnel: [w497 w504 w511 w518 w523 w528 w533] -> w477
              tunnel: [T4."水样测试" ("测量模式") w501 T4."跨度核查" ("测量模式") T4."零点核查" ("测量模式") T4."加标回收" ("测量模式") w527 T4."平行样测试" ("测量模式")] -> w469
              tunnel: w467 -> [_ w503 w509 w516 _ _ _]
              tunnel: [_ w502 w508 w515 _ _ _] -> w476
              tunnel: w462 -> [_ _ _ _ _ w527 _]
              tunnel: w461 -> [_ w501 _ _ _ _ _]
              frame "水样测试", Default {
                n144 = Unbundle By Name(w500) -> ("水样数据时间"=w499:timestamp, "水样实测值"=w498:sgl, "水样数据标识"=w497:string)
              }
              frame "标样核查" {
                n145 = Unbundle By Name(w507) -> ("标样数据时间"=w506:timestamp, "标样实测值"=w505:sgl, "标样数据标识"=w504:string)
                n146 = Unbundle By Name(w503) -> ("亚硝氮标准液标准浓度"=w502:dbl)
              }
              frame "跨度核查" {
                n147 = Unbundle By Name(w514) -> ("跨度核查数据时间"=w513:timestamp, "跨度核查实测值"=w512:sgl, "跨度核查数据标识"=w511:string)
                n148 = Unbundle By Name(w509) -> ("亚硝氮跨度标准液浓度"=w508:dbl)
              }
              frame "零点核查" {
                n149 = Unbundle By Name(w521) -> ("零点核查数据时间"=w520:timestamp, "零点核查实测值"=w519:sgl, "零点核查数据标识"=w518:string)
                n150 = Unbundle By Name(w516) -> ("亚硝氮零点标准液浓度"=w515:dbl)
              }
              frame "加标回收" {
                n151 = Unbundle By Name(w526) -> ("加标回收数据时间"=w525:timestamp, "加标回收实测值"=w524:sgl, "加标回收数据标识"=w523:string)
              }
              frame "空白测试" {
                n152 = Unbundle By Name(w531) -> ("空白数据时间"=w530:timestamp, "空白实测值"=w529:sgl, "空白数据标识"=w528:string)
              }
              frame "平行样" {
                n153 = Unbundle By Name(w536) -> ("平行样数据时间"=w535:timestamp, "平行样实测值"=w534:sgl, "平行样数据标识"=w533:string)
              }
            }
            n154 = Unbundle By Name(w467) -> ("亚硝氮跨度值"=w466:dbl)
            n155 = And(x=w473, y=u16 255) -> (x .and. y?=w474:u16)
            n156 = case shown="0, 默认" w474 {
              tunnel: ["低量程" ("格式字符串") "高量程" ("格式字符串")] -> w472
              frame 0, Default {
              }
              frame 1 {
              }
            }
            n157 = global read "VAR总磷总氮全局变量.vi" "序列号"() -> (w471:string)
            n158 = Bundle By Name(cluster=w468, "时间标识"=w479, "监测值"=w478, "数据标识"=w477, "测量模式"=w469, "单位"=w493, "因子编码"=w492, "标样参考值"=w476, "F0"=w491, "F1"=w490, "F2"=w489, "F3"=w488, "F4"=w487, "F5"=w486, "F6"=w485, "F7"=w484, "X"=w483, "温度"=w482, "湿度"=w481, "量程标识"=w472, "SN"=w471, "数据标记表"=w470, "跨度值"=w466, "X1"=w459) -> (w464:T2)
            n159 = global read "VAR总磷总氮全局变量.vi" "亚硝氮关键参数"() -> (w460:T10)
            n160 = call "总磷氨氮插入数据.vi"("table"=w463, "关键参数"=w460, "data"=w464) -> ()  [unwired: 12 in, 1 out]
          }
          frame 7 {
            n161 = Unbundle By Name(w543) -> ("单位"=w571:u16, "因子编码"=w570:u32, "F0"=w569:sgl, "F1"=w568:sgl, "F2"=w567:sgl, "F3"=w566:sgl, "F4"=w565:sgl, "F5"=w564:sgl, "F6"=w563:sgl, "F7"=w562:sgl, "X值"=w561:sgl, "温度"=w560:sgl, "湿度"=w559:sgl, "fidrange"=w551:u16, "X1值"=w537:sgl)  [unwired: 1 out]
            n162 = global read "总磷总氮断电保存全局变量.vi" "质控参数设置"() -> (w545:T9)
            n163 = case shown="\"空白测试\"" w558 {
              tunnel: w543 -> [w578 w585 w592 w599 w604 w609 w614]
              tunnel: [w577 w584 w591 w598 w603 w608 w613] -> w557
              tunnel: [w576 w583 w590 w597 w602 w607 w612] -> w556
              tunnel: [w575 w582 w589 w596 w601 w606 w611] -> w555
              tunnel: [T4."水样测试" ("测量模式") w579 T4."跨度核查" ("测量模式") T4."零点核查" ("测量模式") T4."加标回收" ("测量模式") w605 T4."平行样测试" ("测量模式")] -> w547
              tunnel: w545 -> [_ w581 w587 w594 _ _ _]
              tunnel: [_ w580 w586 w593 _ _ _] -> w554
              tunnel: w540 -> [_ w579 _ _ _ _ _]
              tunnel: w539 -> [_ _ _ _ _ w605 _]
              frame "水样测试", Default {
                n164 = Unbundle By Name(w578) -> ("水样数据时间"=w577:timestamp, "水样实测值"=w576:sgl, "水样数据标识"=w575:string)
              }
              frame "标样核查" {
                n165 = Unbundle By Name(w585) -> ("标样数据时间"=w584:timestamp, "标样实测值"=w583:sgl, "标样数据标识"=w582:string)
                n166 = Unbundle By Name(w581) -> ("硅酸盐标准液标准浓度"=w580:dbl)
              }
              frame "跨度核查" {
                n167 = Unbundle By Name(w592) -> ("跨度核查数据时间"=w591:timestamp, "跨度核查实测值"=w590:sgl, "跨度核查数据标识"=w589:string)
                n168 = Unbundle By Name(w587) -> ("硅酸盐跨度标准液浓度"=w586:dbl)
              }
              frame "零点核查" {
                n169 = Unbundle By Name(w599) -> ("零点核查数据时间"=w598:timestamp, "零点核查实测值"=w597:sgl, "零点核查数据标识"=w596:string)
                n170 = Unbundle By Name(w594) -> ("硅酸盐零点标准液浓度"=w593:dbl)
              }
              frame "加标回收" {
                n171 = Unbundle By Name(w604) -> ("加标回收数据时间"=w603:timestamp, "加标回收实测值"=w602:sgl, "加标回收数据标识"=w601:string)
              }
              frame "空白测试" {
                n172 = Unbundle By Name(w609) -> ("空白数据时间"=w608:timestamp, "空白实测值"=w607:sgl, "空白数据标识"=w606:string)
              }
              frame "平行样" {
                n173 = Unbundle By Name(w614) -> ("平行样数据时间"=w613:timestamp, "平行样实测值"=w612:sgl, "平行样数据标识"=w611:string)
              }
            }
            n174 = Unbundle By Name(w545) -> ("硅酸盐跨度值"=w544:dbl)
            n175 = And(x=w551, y=u16 255) -> (x .and. y?=w552:u16)
            n176 = case shown="0, 默认" w552 {
              tunnel: ["低量程" ("格式字符串") "高量程" ("格式字符串")] -> w550
              frame 0, Default {
              }
              frame 1 {
              }
            }
            n177 = global read "VAR总磷总氮全局变量.vi" "序列号"() -> (w549:string)
            n178 = Bundle By Name(cluster=w546, "时间标识"=w557, "监测值"=w556, "数据标识"=w555, "测量模式"=w547, "单位"=w571, "因子编码"=w570, "标样参考值"=w554, "F0"=w569, "F1"=w568, "F2"=w567, "F3"=w566, "F4"=w565, "F5"=w564, "F6"=w563, "F7"=w562, "X"=w561, "温度"=w560, "湿度"=w559, "量程标识"=w550, "SN"=w549, "数据标记表"=w548, "跨度值"=w544, "X1"=w537) -> (w542:T2)
            n179 = global read "VAR总磷总氮全局变量.vi" "硅酸盐关键参数"() -> (w538:T10)
            n180 = call "总磷氨氮插入数据.vi"("table"=w541, "关键参数"=w538, "data"=w542) -> ()  [unwired: 12 in, 1 out]
          }
          frame 8 {
            n181 = Unbundle By Name(w621) -> ("单位"=w649:u16, "因子编码"=w648:u32, "F0"=w647:sgl, "F1"=w646:sgl, "F2"=w645:sgl, "F3"=w644:sgl, "F4"=w643:sgl, "F5"=w642:sgl, "F6"=w641:sgl, "F7"=w640:sgl, "X值"=w639:sgl, "温度"=w638:sgl, "湿度"=w637:sgl, "fidrange"=w629:u16, "X1值"=w615:sgl)  [unwired: 1 out]
            n182 = global read "总磷总氮断电保存全局变量.vi" "质控参数设置"() -> (w623:T9)
            n183 = case shown="\"标样核查\"" w636 {
              tunnel: w621 -> [w656 w663 w670 w677 w682 w687 w692]
              tunnel: [w655 w662 w669 w676 w681 w686 w691] -> w635
              tunnel: [w654 w661 w668 w675 w680 w685 w690] -> w634
              tunnel: [w653 w660 w667 w674 w679 w684 w689] -> w633
              tunnel: [T4."水样测试" ("测量模式") w657 T4."跨度核查" ("测量模式") T4."零点核查" ("测量模式") T4."加标回收" ("测量模式") w683 T4."平行样测试" ("测量模式")] -> w625
              tunnel: w623 -> [_ w659 w665 w672 _ _ _]
              tunnel: [_ w658 w664 w671 _ _ _] -> w632
              tunnel: w618 -> [_ _ _ _ _ w683 _]
              tunnel: w617 -> [_ w657 _ _ _ _ _]
              frame "水样测试", Default {
                n184 = Unbundle By Name(w656) -> ("水样数据时间"=w655:timestamp, "水样实测值"=w654:sgl, "水样数据标识"=w653:string)
              }
              frame "标样核查" {
                n185 = Unbundle By Name(w663) -> ("标样数据时间"=w662:timestamp, "标样实测值"=w661:sgl, "标样数据标识"=w660:string)
                n186 = Unbundle By Name(w659) -> ("硫化物标准液标准浓度"=w658:dbl)
              }
              frame "跨度核查" {
                n187 = Unbundle By Name(w670) -> ("跨度核查数据时间"=w669:timestamp, "跨度核查实测值"=w668:sgl, "跨度核查数据标识"=w667:string)
                n188 = Unbundle By Name(w665) -> ("硫化物跨度标准液浓度"=w664:dbl)
              }
              frame "零点核查" {
                n189 = Unbundle By Name(w677) -> ("零点核查数据时间"=w676:timestamp, "零点核查实测值"=w675:sgl, "零点核查数据标识"=w674:string)
                n190 = Unbundle By Name(w672) -> ("硫化物零点标准液浓度"=w671:dbl)
              }
              frame "加标回收" {
                n191 = Unbundle By Name(w682) -> ("加标回收数据时间"=w681:timestamp, "加标回收实测值"=w680:sgl, "加标回收数据标识"=w679:string)
              }
              frame "空白测试" {
                n192 = Unbundle By Name(w687) -> ("空白数据时间"=w686:timestamp, "空白实测值"=w685:sgl, "空白数据标识"=w684:string)
              }
              frame "平行样" {
                n193 = Unbundle By Name(w692) -> ("平行样数据时间"=w691:timestamp, "平行样实测值"=w690:sgl, "平行样数据标识"=w689:string)
              }
            }
            n194 = Unbundle By Name(w623) -> ("硫化物跨度值"=w622:dbl)
            n195 = And(x=w629, y=u16 255) -> (x .and. y?=w630:u16)
            n196 = case shown="0, 默认" w630 {
              tunnel: ["低量程" ("格式字符串") "高量程" ("格式字符串")] -> w628
              frame 0, Default {
              }
              frame 1 {
              }
            }
            n197 = global read "VAR总磷总氮全局变量.vi" "序列号"() -> (w627:string)
            n198 = Bundle By Name(cluster=w624, "时间标识"=w635, "监测值"=w634, "数据标识"=w633, "测量模式"=w625, "单位"=w649, "因子编码"=w648, "标样参考值"=w632, "F0"=w647, "F1"=w646, "F2"=w645, "F3"=w644, "F4"=w643, "F5"=w642, "F6"=w641, "F7"=w640, "X"=w639, "温度"=w638, "湿度"=w637, "量程标识"=w628, "SN"=w627, "数据标记表"=w626, "跨度值"=w622, "X1"=w615) -> (w620:T2)
            n199 = global read "VAR总磷总氮全局变量.vi" "硫化物关键参数"() -> (w616:T10)
            n200 = call "总磷氨氮插入数据.vi"("table"=w619, "关键参数"=w616, "data"=w620) -> ()  [unwired: 12 in, 1 out]
          }
          frame 22 {
            n201 = Unbundle By Name(w698) -> ("单位"=w727:u16, "因子编码"=w726:u32, "F0"=w725:sgl, "F1"=w724:sgl, "F2"=w723:sgl, "F3"=w722:sgl, "F4"=w721:sgl, "F5"=w720:sgl, "F6"=w719:sgl, "F7"=w718:sgl, "X值"=w717:sgl, "温度"=w716:sgl, "湿度"=w715:sgl, "fidrange"=w707:u16, "X1值"=w693:sgl)  [unwired: 1 out]
            n202 = global read "总磷总氮断电保存全局变量.vi" "质控参数设置"() -> (w700:T9)
            n203 = case shown="\"标样核查\"" w714 {
              tunnel: w698 -> [w734 w741 w748 w755 w760 w765 w770]
              tunnel: [w733 w740 w747 w754 w759 w764 w769] -> w713
              tunnel: [w732 w739 w746 w753 w758 w763 w768] -> w712
              tunnel: [w731 w738 w745 w752 w757 w762 w767] -> w711
              tunnel: [T4."水样测试" ("测量模式") w735 T4."跨度核查" ("测量模式") T4."零点核查" ("测量模式") T4."加标回收" ("测量模式") w761 T4."平行样测试" ("测量模式")] -> w703
              tunnel: w700 -> [_ w737 w743 w750 _ _ _]
              tunnel: [_ w736 w742 w749 _ _ _] -> w710
              tunnel: w696 -> [_ _ _ _ _ w761 _]
              tunnel: w695 -> [_ w735 _ _ _ _ _]
              frame "水样测试", Default {
                n204 = Unbundle By Name(w734) -> ("水样数据时间"=w733:timestamp, "水样实测值"=w732:sgl, "水样数据标识"=w731:string)
              }
              frame "标样核查" {
                n205 = Unbundle By Name(w741) -> ("标样数据时间"=w740:timestamp, "标样实测值"=w739:sgl, "标样数据标识"=w738:string)
                n206 = Unbundle By Name(w737) -> ("COD标准液标准浓度"=w736:dbl)
              }
              frame "跨度核查" {
                n207 = Unbundle By Name(w748) -> ("跨度核查数据时间"=w747:timestamp, "跨度核查实测值"=w746:sgl, "跨度核查数据标识"=w745:string)
                n208 = Unbundle By Name(w743) -> ("COD跨度标准液浓度"=w742:dbl)
              }
              frame "零点核查" {
                n209 = Unbundle By Name(w755) -> ("零点核查数据时间"=w754:timestamp, "零点核查实测值"=w753:sgl, "零点核查数据标识"=w752:string)
                n210 = Unbundle By Name(w750) -> ("COD零点标准液浓度"=w749:dbl)
              }
              frame "加标回收" {
                n211 = Unbundle By Name(w760) -> ("加标回收数据时间"=w759:timestamp, "加标回收实测值"=w758:sgl, "加标回收数据标识"=w757:string)
              }
              frame "空白测试" {
                n212 = Unbundle By Name(w765) -> ("空白数据时间"=w764:timestamp, "空白实测值"=w763:sgl, "空白数据标识"=w762:string)
              }
              frame "平行样" {
                n213 = Unbundle By Name(w770) -> ("平行样数据时间"=w769:timestamp, "平行样实测值"=w768:sgl, "平行样数据标识"=w767:string)
              }
            }
            n214 = Unbundle By Name(w700) -> ("COD跨度值"=w699:dbl)
            n215 = And(x=w707, y=u16 255) -> (x .and. y?=w708:u16)
            n216 = case shown="0, 默认" w708 {
              tunnel: ["低量程" ("格式字符串") "高量程" ("格式字符串")] -> w706
              frame 0, Default {
              }
              frame 1 {
              }
            }
            n217 = global read "VAR总磷总氮全局变量.vi" "序列号"() -> (w705:string)
            n218 = Bundle By Name(cluster=w702, "时间标识"=w713, "监测值"=w712, "数据标识"=w711, "测量模式"=w703, "单位"=w727, "因子编码"=w726, "标样参考值"=w710, "F0"=w725, "F1"=w724, "F2"=w723, "F3"=w722, "F4"=w721, "F5"=w720, "F6"=w719, "F7"=w718, "X"=w717, "温度"=w716, "湿度"=w715, "量程标识"=w706, "SN"=w705, "数据标记表"=w704, "跨度值"=w699, "X1"=w693) -> (w701:T2)
            n219 = global read "VAR总磷总氮全局变量.vi" "CODcr关键参数"() -> (w694:T10)
            n220 = call "总磷氨氮插入数据.vi"("table"=w697, "关键参数"=w694, "data"=w701) -> ()  [unwired: 12 in, 1 out]
          }
          frame 50 {
            n221 = Unbundle By Name(w776) -> ("单位"=w805:u16, "因子编码"=w804:u32, "F0"=w803:sgl, "F1"=w802:sgl, "F2"=w801:sgl, "F3"=w800:sgl, "F4"=w799:sgl, "F5"=w798:sgl, "F6"=w797:sgl, "F7"=w796:sgl, "X值"=w795:sgl, "温度"=w794:sgl, "湿度"=w793:sgl, "fidrange"=w785:u16, "X1值"=w771:sgl)  [unwired: 1 out]
            n222 = global read "总磷总氮断电保存全局变量.vi" "质控参数设置"() -> (w778:T9)
            n223 = Unbundle By Name(w778) -> ("氟化物跨度值"=w777:dbl)
            n224 = case shown="\"平行样\"" w792 {
              tunnel: w776 -> [w812 w819 w826 w833 w838 w843 w848]
              tunnel: [w811 w818 w825 w832 w837 w842 w847] -> w791
              tunnel: [w810 w817 w824 w831 w836 w841 w846] -> w790
              tunnel: [w809 w816 w823 w830 w835 w840 w845] -> w789
              tunnel: [T4."水样测试" ("测量模式") w813 T4."跨度核查" ("测量模式") T4."零点核查" ("测量模式") T4."加标回收" ("测量模式") w839 T4."平行样测试" ("测量模式")] -> w781
              tunnel: w778 -> [_ w815 w821 w828 _ _ _]
              tunnel: [_ w814 w820 w827 _ _ _] -> w788
              tunnel: w774 -> [_ _ _ _ _ w839 _]
              tunnel: w773 -> [_ w813 _ _ _ _ _]
              frame "水样测试", Default {
                n225 = Unbundle By Name(w812) -> ("水样数据时间"=w811:timestamp, "水样实测值"=w810:sgl, "水样数据标识"=w809:string)
              }
              frame "标样核查" {
                n226 = Unbundle By Name(w815) -> ("氟化物标准液标准浓度"=w814:dbl)
                n227 = Unbundle By Name(w819) -> ("标样数据时间"=w818:timestamp, "标样实测值"=w817:sgl, "标样数据标识"=w816:string)
              }
              frame "跨度核查" {
                n228 = Unbundle By Name(w821) -> ("氟化物跨度标准液浓度"=w820:dbl)
                n229 = Unbundle By Name(w826) -> ("跨度核查数据时间"=w825:timestamp, "跨度核查实测值"=w824:sgl, "跨度核查数据标识"=w823:string)
              }
              frame "零点核查" {
                n230 = Unbundle By Name(w828) -> ("氟化物零点标准液浓度"=w827:dbl)
                n231 = Unbundle By Name(w833) -> ("零点核查数据时间"=w832:timestamp, "零点核查实测值"=w831:sgl, "零点核查数据标识"=w830:string)
              }
              frame "加标回收" {
                n232 = Unbundle By Name(w838) -> ("加标回收数据时间"=w837:timestamp, "加标回收实测值"=w836:sgl, "加标回收数据标识"=w835:string)
              }
              frame "空白测试" {
                n233 = Unbundle By Name(w843) -> ("空白数据时间"=w842:timestamp, "空白实测值"=w841:sgl, "空白数据标识"=w840:string)
              }
              frame "平行样" {
                n234 = Unbundle By Name(w848) -> ("平行样数据时间"=w847:timestamp, "平行样实测值"=w846:sgl, "平行样数据标识"=w845:string)
              }
            }
            n235 = And(x=w785, y=u16 255) -> (x .and. y?=w786:u16)
            n236 = case shown="1" w786 {
              tunnel: ["低量程" ("格式字符串") "高量程" ("格式字符串")] -> w784
              frame 0, Default {
              }
              frame 1 {
              }
            }
            n237 = global read "VAR总磷总氮全局变量.vi" "序列号"() -> (w783:string)
            n238 = Bundle By Name(cluster=w780, "时间标识"=w791, "监测值"=w790, "数据标识"=w789, "测量模式"=w781, "单位"=w805, "因子编码"=w804, "标样参考值"=w788, "F0"=w803, "F1"=w802, "F2"=w801, "F3"=w800, "F4"=w799, "F5"=w798, "F6"=w797, "F7"=w796, "X"=w795, "温度"=w794, "湿度"=w793, "量程标识"=w784, "SN"=w783, "数据标记表"=w782, "跨度值"=w777, "X1"=w771) -> (w779:T2)
            n239 = global read "VAR总磷总氮全局变量.vi" "氟化物关键参数"() -> (w772:T10)
            n240 = call "总磷氨氮插入数据.vi"("table"=w775, "关键参数"=w772, "data"=w779) -> ()  [unwired: 12 in, 1 out]
          }
        }
      }
    }
  }
